vi "Initialize Custom Device.vi"(8 "error in":errorcluster, 11 "Ballard ARINC 429 ref":T1=18446744073709551615 format="%.0x") -> (0 "error out":errorcluster, 3 "Ballard ARINC 429 ref out":T1 format="%.0x")   [LabVIEW 2020, in "Ballard ARINC 429 Scripting.lvlib"]
uses:
  Ballard ARINC 429 Scripting.lvlib
  <vilib>/NI VeriStand/Custom Device API/Custom Device Item Ref.ctl
  <vilib>/NI VeriStand/Custom Device API/Custom Device API.lvlib
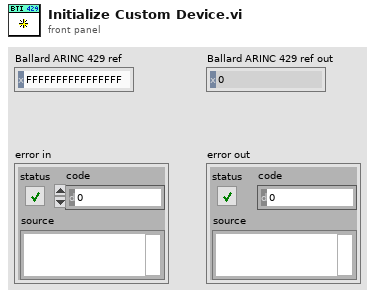
[diagram p1: front panel]
types:
  T1 = typedef "Custom Device API.lvlib/Custom Device Item Ref.ctl" = u64
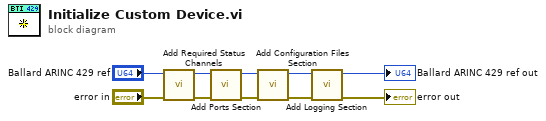
[diagram p0: block diagram]
diagram:
  n1 = call "Add Required Status Channels.vi"("error in"="error in", "custom device ref"="Ballard ARINC 429 ref") -> ("error out"=w8:errorcluster, "custom device ref out"=w7:T1)  [unwired: 7 in, 1 out]
  n2 = call "Add Ports Section.vi"("error in"=w8, "custom device ref"=w7) -> ("error out"=w10:errorcluster, "custom device ref out"=w9:T1)  [unwired: 7 in, 1 out]
  n3 = call "Add Configuration Files Section.vi"("error in"=w10, "Custom device Ref"=w9) -> ("error out"=w3:errorcluster, "Custom device Ref out"=w4:T1)  [unwired: 7 in, 1 out]
  n4 = call "Add Logging Section.vi"("error in"=w3, "custom device ref"=w4) -> ("error out"=→"error out":errorcluster, "custom device ref out"=→"Ballard ARINC 429 ref out":T1)  [unwired: 7 in, 1 out]
